vi "Tag Expr Test.vi"() -> ()   [LabVIEW 2018]
uses:
  Tag/Tag.lvclass/Tag.ctl
  Tag Expr/Tag Expr.lvclass
  C:/Program Files (x86)/National Instruments/LabVIEW 2018/vi.lib/LAVA/muParser/mupExpr/mupExpr.lvclass
  Tag Expr/Tag Expr.lvclass/Tag Expr.ctl
  <vilib>/LAVA/muParser/mupExpr/mupExpr.lvclass/mupExpr.ctl
  ca4c7cba-ec31-482d-bafe-c426c48bc65d.vi
  94d3df27-bc47-4a3a-955d-f026f475c6e0.vi
  <vilib>/LAVA/muParser/mupExpr/Eval.vi
  <vilib>/LAVA/muParser/mupExpr/Eval_SglRes.vi
  CVT Expr/Lookup CVT Values.vi
  <vilib>/LAVA/muParser/mupLib/mupEval.vi
  CVT Expr/Lookup CVT Values.vi/7ca61f51-c808-43da-a40e-90d99acaf134.vi
  <vilib>/LAVA/muParser/mupExpr/Set_Var_Value.vi
  <vilib>/LAVA/muParser/mupExpr/Set_MultiVar_Value.vi
  <vilib>/LAVA/muParser/mupLib/mupCheckError.vi
  <vilib>/LAVA/muParser/mupLib/mupLibPath.vi
  Tag/Read Value.vi
  Tag/Read Timestamp.vi
  <vilib>/LAVA/muParser/mupExpr/SetVarVal.vi
  <vilib>/LAVA/muParser/mupLib/mupSetVarValue.vi
  Tag/Set Properties from Initial.vi
  Core/Add Tag.vi
  <vilib>/Utility/error.llb/Error Cluster From Error Code.vi
  Tag/Tag.lvclass
panel:
  out "Boolear Result":bool
  out "Result":dbl format="%#_13g"
  in  "Expression":string="50/test2+23+test1"
  out "error out":errorcluster
  out "Variable Names":string[](array[string])
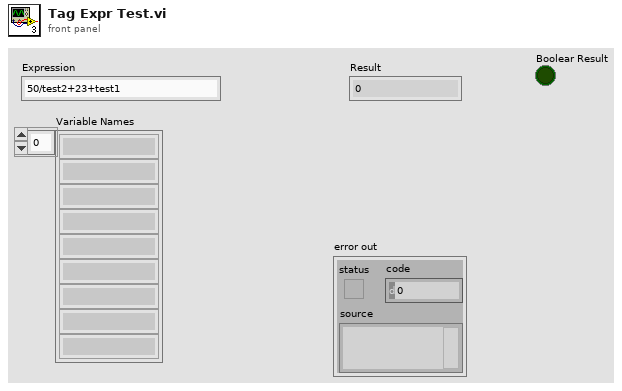
[diagram p1: front panel]
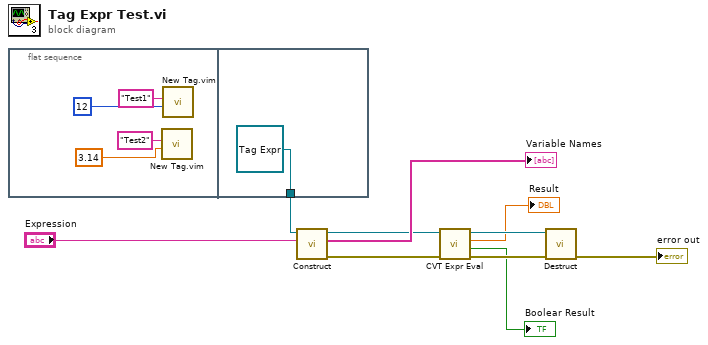
[diagram p0: block diagram]
diagram:
  n1 = flat-sequence {
    tunnel: [refnum<class "Tag Expr.lvclass"> refnum ("CVT Engine:CVT Expr.lvclass")] -> w1
    frame #0 {
      n2 = call "New Tag.vim"("Initial Value"=3.14, "Tag Name"="Test2" ("Name")) -> ()  [unwired: 8 in, 2 out]
      n3 = call "New Tag.vim"("Initial Value"=12, "Tag Name"="Test1" ("Name")) -> ()  [unwired: 8 in, 2 out]
    }
    frame #1 {
    }
  }
  n4 = call-dynamic "Construct.vi"("Expression"="Expression", "muExpr in"=w1) -> ("error out"=w5:errorcluster, "Variable Names"=→"Variable Names":string[], "CVT Expr out"=w8:refnum<class "Tag Expr.lvclass">)  [unwired: 6 in, 1 out]
  n5 = call "CVT Expr Eval.vi"("error in (no error)"=w5, "CVT Expr in"=w8) -> ("error out"=w6:errorcluster, "Boolear Result"=→"Boolear Result":bool, "Result"=→"Result":dbl, "CVT Expr out"=w7:refnum<class "Tag Expr.lvclass">)  [unwired: 6 in]
  n6 = call-dynamic "Destruct.vi"("error in (no error)"=w6, "muExpr in"=w7) -> ("error out"=→"error out":errorcluster)  [unwired: 9 in]
